vi "WashDisplay_QueueOperations_FGV.vi"(8 "error in":errorcluster, 10 "Data In":T1, 11 "Action":T3) -> (0 "error out":errorcluster, 1 "#elements in queue":i32, 2 "elements in queue":T1[](array[typedef]), 3 "queue ref":refnum<queue>)   [LabVIEW 2019]
uses:
  #typedef_Queue_enum.ctl
  #typedef_Data_WashDisplay.ctl
  #typedef_WashDisplay_Action_enum.ctl
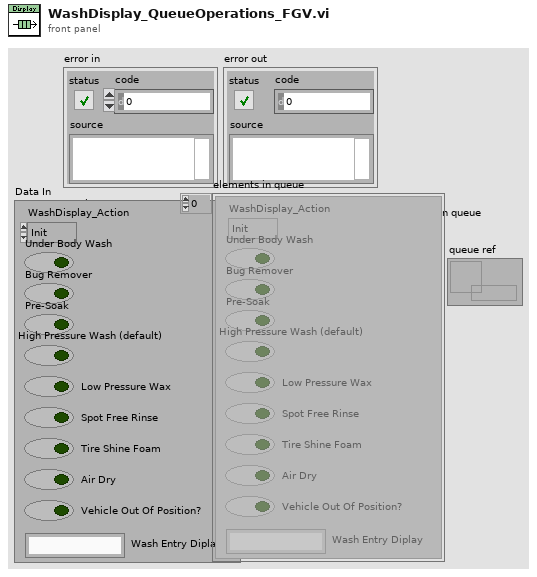
[diagram p1: front panel]
types:
  T1 = typedef "#typedef_Data_WashDisplay.ctl" = cluster{"WashDisplay_Action":T2, "Under Body Wash":bool, "Bug Remover":bool, "Pre-Soak":bool, "High Pressure Wash (default)":bool, "Low Pressure Wax":bool, "Spot Free Rinse":bool, "Tire Shine Foam":bool, "Air Dry":bool, "Vehicle Out Of Position?":bool, "Wash Entry Diplay":string}
  T2 = typedef "#typedef_WashDisplay_Action_enum.ctl" = enum16{"Init", "ERROR_DEFAULT", "Idle", "Update FP", "Close", "Error_Handler", "Exit"}
  T3 = typedef "#typedef_Queue_enum.ctl" = enum16{"ERROR_default", "Obtain", "Enqueue", "GetStatus", "Flush", "Release"}
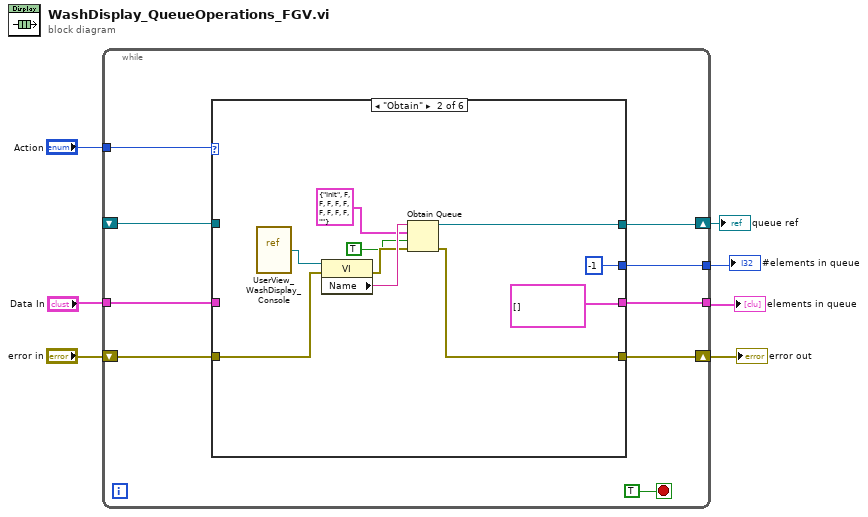
[diagram p0: block diagram]
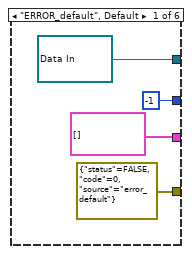
[diagram p2: hidden frame]
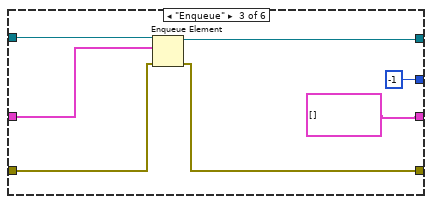
[diagram p3: hidden frame]
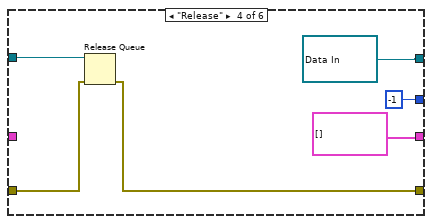
[diagram p4: hidden frame]
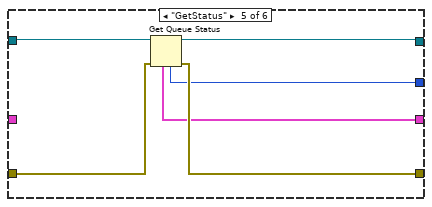
[diagram p5: hidden frame]
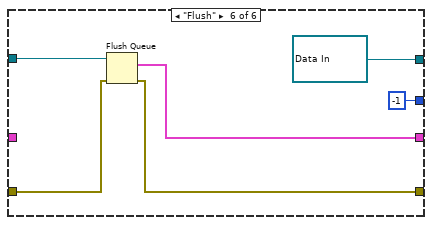
[diagram p6: hidden frame]
diagram:
  n1 = while {
    tunnel: "Action" -> [w15]
    tunnel: "Data In" -> [w13]
    tunnel: [w10] -> w1
    shift-right: [w11] -> w4
    shift-left: _ -> [w9]
    shift-right: [w12] -> w5
    shift-left: "error in" -> [w14]
    tunnel: [w8] -> w2
    stop <- TRUE stop-if-true
    n2 = case shown="\"Obtain\"" w15 {
      tunnel: w14 -> [_ w30 w35 w42 w46 w54]
      tunnel: w13 -> [_ _ w36 _ _ _]
      tunnel: [errorcluster {"status"=FALSE, "code"=0, "source"="error_default"} ("error out") w27 w34 w41 w47 w53] -> w12
      tunnel: [refnum<queue> refnum ("queue out") w26 w33 refnum<queue> refnum ("queue out") w48 refnum<queue> refnum ("queue out")] -> w11
      tunnel: [-1 ("# elements in queue") -1 ("#elements in queue") -1 ("#elements in queue") -1 ("# elements in queue") w44 -1 ("# elements in queue")] -> w10
      tunnel: w9 -> [_ _ w37 w43 w49 w55]
      tunnel: [T1[] [] T1[] [] T1[] [] T1[] [] w45 w52] -> w8
      frame "ERROR_default", Default {
      }
      frame "Obtain" {
        n3 = vi-ref "UserView_WashDisplay_Console.vi"() -> (w23:refnum<vi>)
        n4 = property class="VI"(reference=w23, error in=w30) -> (error out=w28:errorcluster, "Name"=w29:string)  [unwired: 1 out]
        n5 = Obtain Queue(name (unnamed)=w29, element data type=T1 {"WashDisplay_Action"=enum."Init", "Under Body Wash"=FALSE, "Bug Remover"=FALSE, "Pre-Soak"=FALSE, "High Pressure Wash (default)"=FALSE, "Low Pressure Wax"=FALSE, "Spot Free Rinse"=FALSE, "Tire Shine Foam"=FALSE, "Air Dry"=FALSE, "Vehicle Out Of Position?"=FALSE, "Wash Entry Diplay"=""} ("Data In"), create if not found? (T)=TRUE, error in (no error)=w28) -> (queue out=w26:refnum<queue>, error out=w27:errorcluster)  [unwired: 1 in, 1 out]
      }
      frame "Enqueue" {
        n6 = Enqueue Element(queue=w37, element=w36, error in (no error)=w35) -> (queue out=w33:refnum<queue>, error out=w34:errorcluster)  [unwired: 1 in, 1 out]
      }
      frame "Release" {
        n7 = Release Queue(queue=w43, error in (no error)=w42) -> (error out=w41:errorcluster)  [unwired: 1 in, 2 out]
      }
      frame "GetStatus" {
        n8 = Get Queue Status(queue=w49, error in (no error)=w46) -> (queue out=w48:refnum<queue>, error out=w47:errorcluster, # elements in queue=w44:i32, elements=w45:T1[])  [unwired: 1 in, 4 out]
      }
      frame "Flush" {
        n9 = Flush Queue(queue=w55, error in (no error)=w54) -> (remaining elements=w52:T1[], error out=w53:errorcluster)  [unwired: 1 out]
      }
    }
  }
  "error out" <- w5
  "#elements in queue" <- w1
  "elements in queue" <- w2
  "queue ref" <- w4
